vi "alltables.vi"() -> ()   [LabVIEW 2017]
uses:
  Beltwatch/BeltWatch 4-2-2-5/BeltWatch Event.ctl
  Beltwatch/BeltWatch 4-2-2-5/BeltWatch Event type.ctl
  Beltwatch/BeltWatch 4-2-2-5/BeltWatch Reading.ctl
  Beltwatch/BeltWatch 4-2-2-5/BeltWatch Alarm Priority.ctl
  Beltwatch/BeltWatch 4-2-2-5/BeltWatch 2D overlay.ctl
  Beltwatch/BeltWatch 4-2-2-5/Overlay mode.ctl
  Beltwatch/BeltWatch 4-2-2-5/Events class.ctl
panel:
  out "Label.Text":string
  out "Element Names":string[](array[string])
  out "Tables":string[](array[string])
  out "xml string":string
  out "data string":string
  in  "Event Out":T1
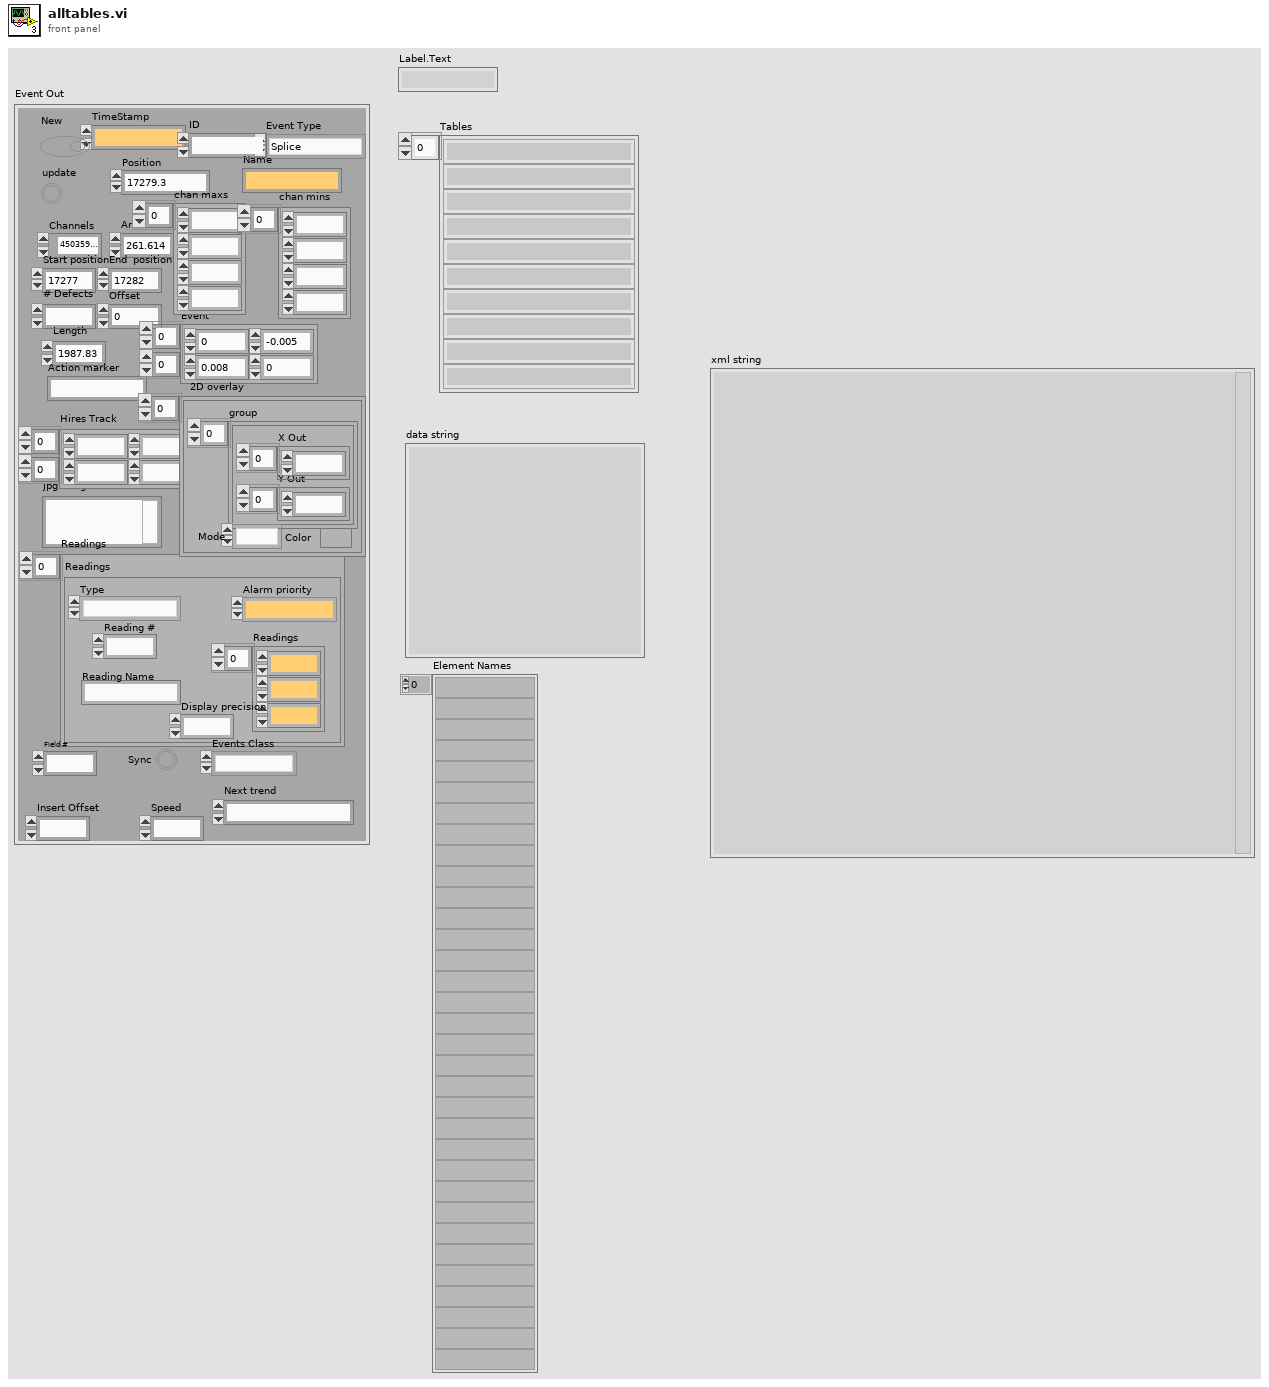
[diagram p1: front panel]
types:
  T1 = typedef "BeltWatch Event.ctl" = cluster{"Position":dbl, "Event Type":T2, "Area":dbl, "Channels":u64, "Start position":dbl, "End  position":dbl, "Name":string, "Offset":dbl, "Length":dbl, "Action marker":string, "Event":dbl[][], "# Defects":i32, "jpg Image":string, "chan maxs":dbl[], "chan mins":dbl[], "TimeStamp":dbl, "Readings":T3[], "ID":u32, "New":bool, "Hires Track":dbl[][], "2D overlay":T5, "update":bool, "Field #":i32, "Events Class":T7, "Sync":bool, "Insert Offset":dbl, "Next trend":dbl, "Speed":dbl}
  T2 = typedef "BeltWatch Event type.ctl" = enum16{"Defect", "Splice", "Break", "Rip", "Track", "Segment", "Belt", "New Splice", "Missing Splice", "None", "Free"}
  T3 = typedef "BeltWatch Reading.ctl" = cluster{"Reading #":i32, "Readings":dbl[], "Reading Name":string, "Type":T2, "Alarm priority":T4, "Display precision":i32}
  T4 = typedef "BeltWatch Alarm Priority.ctl" = enum16{"No Alarm", "High", "Medium", "Low"}
  T5 = typedef "BeltWatch 2D overlay.ctl" = cluster{"group":cluster{"X Out":sgl[], "Y Out":sgl[]}[], "Color ":u32, "Mode":T6}[]
  T6 = typedef "Overlay mode.ctl" = enum16{"Line", "point", "Box", "Oval", "Numbannotation"}
  T7 = typedef "Events class.ctl" = enum16{"Reference", "Inspection", "New", "Tramp", "Align", "Ready"}
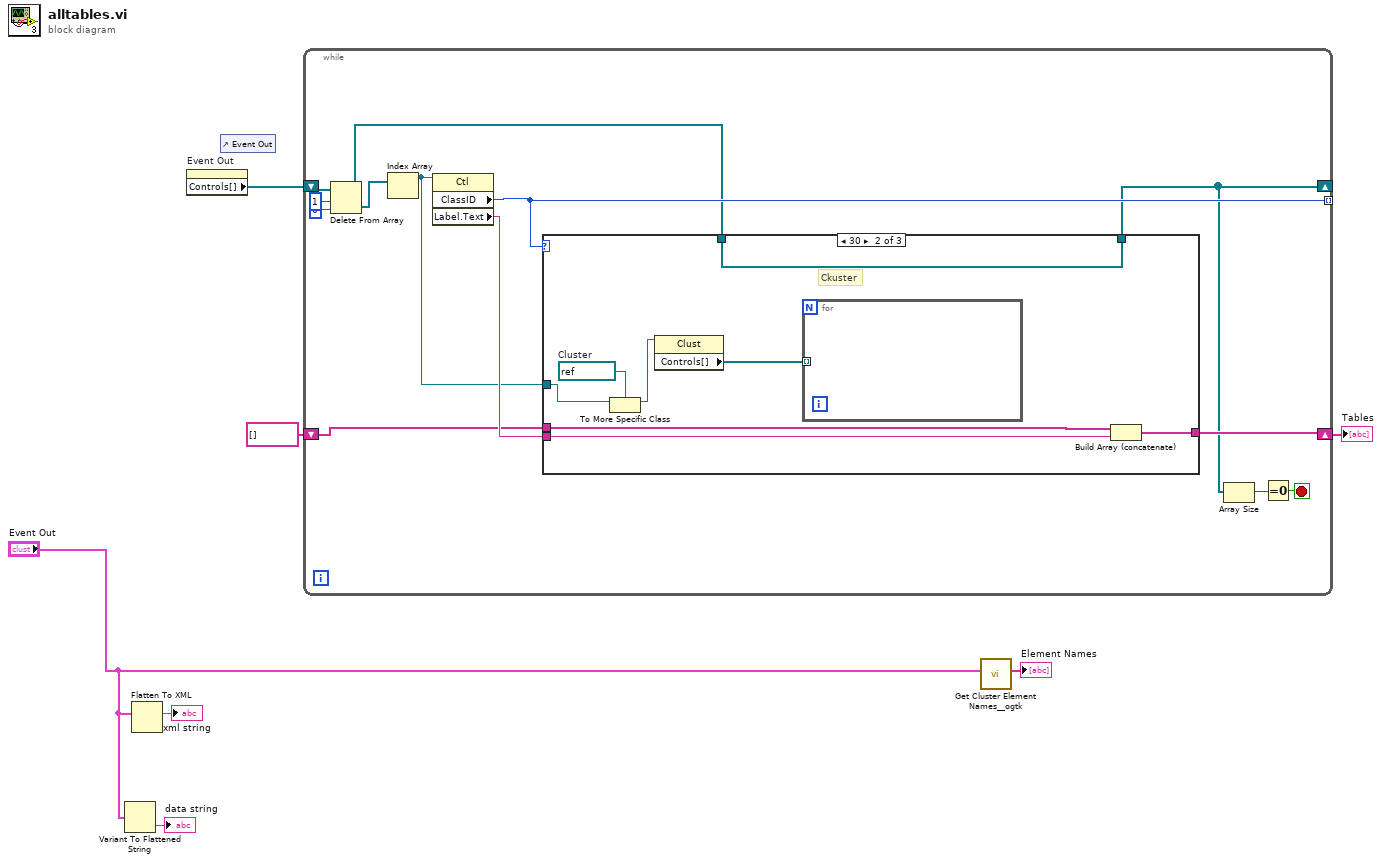
[diagram p0: block diagram]
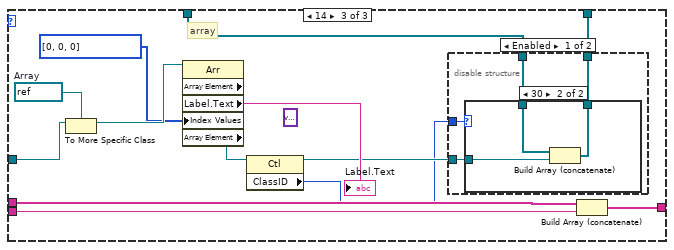
[diagram p3: hidden frame]
diagram:
  n1 = Variant To Flattened String(Variant="Event Out") -> (data string=→"data string":string)  [unwired: 1 out]
  n2 = Flatten To XML(anything="Event Out") -> (xml string=→"xml string":string)
  n3 = property on="Event Out" class="Clust (strict)"() -> ("Controls[]"=w3:refnum<vi>[])  [unwired: 2 in, 2 out]
  n4 = control-ref of="Event Out"() -> ()  [unwired: 1 out]
  n5 = while {
    tunnel: [w20] -> _ mode=indexing
    shift-right: [w18] -> w4
    shift-left: string[] [] -> [w17]
    shift-right: [w11] -> _
    shift-left: w3 -> [w16]
    stop <- w9 stop-if-true
    n6 = Delete From Array(array=w16, length=1, index=0) -> (deleted portion=w12:refnum<vi>[], array with subset deleted=w13:refnum<vi>[])
    n7 = Index Array(array=w12) -> (element=w8:refnum<vi>)  [unwired: 1 in]
    n8 = property class="Ctl"(reference=w8) -> ("ClassID"=w20:u32, "Label.Text"=w19:string)  [unwired: 1 in, 2 out]
    n9 = case shown="30" w20 {
      tunnel: w19 -> [_ w30 w43]
      tunnel: [w22 w29 w42] -> w18
      tunnel: w17 -> [w22 w28 w41]
      tunnel: w13 -> [w21 w27 w40]
      tunnel: [w21 w27 w39] -> w11
      tunnel: w8 -> [_ w25 w36]
      frame 0, Default {
      }
      frame 30 {
        w26 = refnum<vi> refnum  # Cluster
        # "Ckuster"
        n10 = To More Specific Class(target class=w26, reference=w25) -> (specific class reference=w24:refnum<vi>)  [unwired: 1 in, 1 out]
        n11 = property class="Clust"(reference=w24) -> ("Controls[]"=w23:refnum<vi>[])  [unwired: 1 in, 2 out]
        n12 = for {
          tunnel: w23 -> [_] mode=indexing
        }
        n13 = Build Array (concatenate)(w28, w30) -> (w29:string[])
      }
      frame 14 {
        w37 = refnum<vi> refnum  # Array
        (unwired) variant ("Value")
        # "array"
        n14 = To More Specific Class(target class=w37, reference=w36) -> (specific class reference=w35:refnum<vi>)  [unwired: 1 in, 1 out]
        n15 = property class="Arr" props=["Array Element", "Label", "Text", "Index Values", "Array Element"](reference=w35, "Index Values"=u32[] [0, 0, 0]) -> ("Label.Text"=→"Label.Text":string, "Array Element"=w33:refnum<vi>)  [unwired: 1 in, 3 out]
        n16 = property class="Ctl"(reference=w33) -> (reference out=w32:refnum<vi>, "ClassID"=w31:u32)  [unwired: 1 in, 1 out]
        n17 = disable-structure shown="Enabled" {
          disable-tunnel: w40 -> [w47 w52]
          disable-tunnel: [w46 w52] -> w39
          disable-tunnel: w32 -> [w45 _]
          disable-tunnel: w31 -> [w44 _]
          frame Enabled {
            n18 = case shown="30" w44 {
              tunnel: w47 -> [w48 w51]
              tunnel: [w48 w50] -> w46
              tunnel: w45 -> [_ w49]
              frame 0, Default {
              }
              frame 30 {
                n19 = Build Array (concatenate)(w51, w49) -> (w50:refnum<vi>[])
              }
            }
          }
          frame Disabled {
          }
        }
        n20 = Build Array (concatenate)(w41, w43) -> (w42:string[])
      }
    }
    n21 = Array Size(array=w11) -> (size(s)=w10:i32)
    n22 = Equal To 0?(x=w10) -> (x = 0?=w9:bool)
  }
  "Tables" <- w4
  n23 = call <userlib>:"Get Cluster Element Names__ogtk.vi"("Cluster"="Event Out") -> ("Element Names"=→"Element Names":string[])  [unwired: 9 in, 1 out]
